vi "Main.vi"(8 "error in":errorcluster, 9 "Error Queue":refnum<queue>, 10 "Controller Queue":refnum<queue>, 11 "Application Events":refnum<user-event>) -> (0 "error out":errorcluster)   [LabVIEW 2020, in "Display Console.lvlib"]
uses:
  Display Console.lvlib
  Controller/Controls/Module Message.ctl
  Controller/Controls/Application Modules.ctl
  Controller/Controls/Application Event Message.ctl
  Controller/Controls/Application Events.ctl
  Controls/Module Loop Data.ctl
  Controller/Controller.lvlib
panel:
  out "Emergency":bool
  out "Door Open":bool
  out "Elevator Direction":cluster{"Up":bool, "Down":bool}
  out "Elevator Location":string
  out "Timing":string
  # "[Covers: UI3] \n[Covers: UI3A] \n[Covers: UI3A1] \n[Covers: UI3A2] \n[Covers: UI3B] \n[Covers: UI3C] \n[Covers: UI3D] \n[Covers: UI3D1] \n[Covers: UI3D2] \n[Covers: UI3E]"
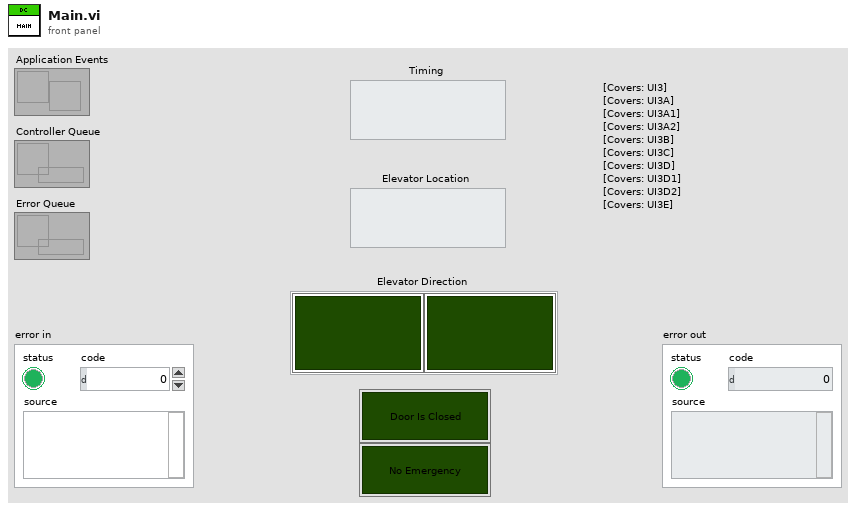
[diagram p1: front panel]
types:
  T1 = typedef "Controller.lvlib/Application Events.ctl" = enum16{"Controller: Initialize", "Controller: Initialize Start And Move State", "Controller: Initialize Analysis State", "Controller: Initialize Continue Travel State", "Controller: Initialize Stop At Floor", "Controller: Initialize Open And Close Door Sequence", "Controller: Initialize No Request Remaining", "Controller: Initialize Emergency Call", "Controller: Initialize Terminate Process", "Controller: Publish State", "UI: Elevator Call", "UI: Broadcast State", "UI: Next Destination Reached", "UI: Timeout Reached", "UI: Emergency Call", "UI: Terminate State", "UI: Door Opened", "UI: Door Closed", "UI: Floor Reached", "UI: Door About To Close"}
  T2 = typedef "Display Console.lvlib/Module Loop Data.ctl" = cluster{"Timing":cluster{"IsTiming?":bool, "Time Target Sec":dbl, "Time Ticks Ms":i32, "Time Ticks Counter":i32, "Timeout Event":T3}, "Is Elevator Travelling?":bool, "Is Elevator opening Door?":bool}
  T3 = typedef "Controller.lvlib/Application Event Message.ctl" = cluster{"Source":T4, "Event":T1, "Data":variant}
  T4 = typedef "Controller.lvlib/Application Modules.ctl" = enum16{"Controller", "User Console", "Display Console", "Sensor Interface", "Configuration Database", "Error Module"}
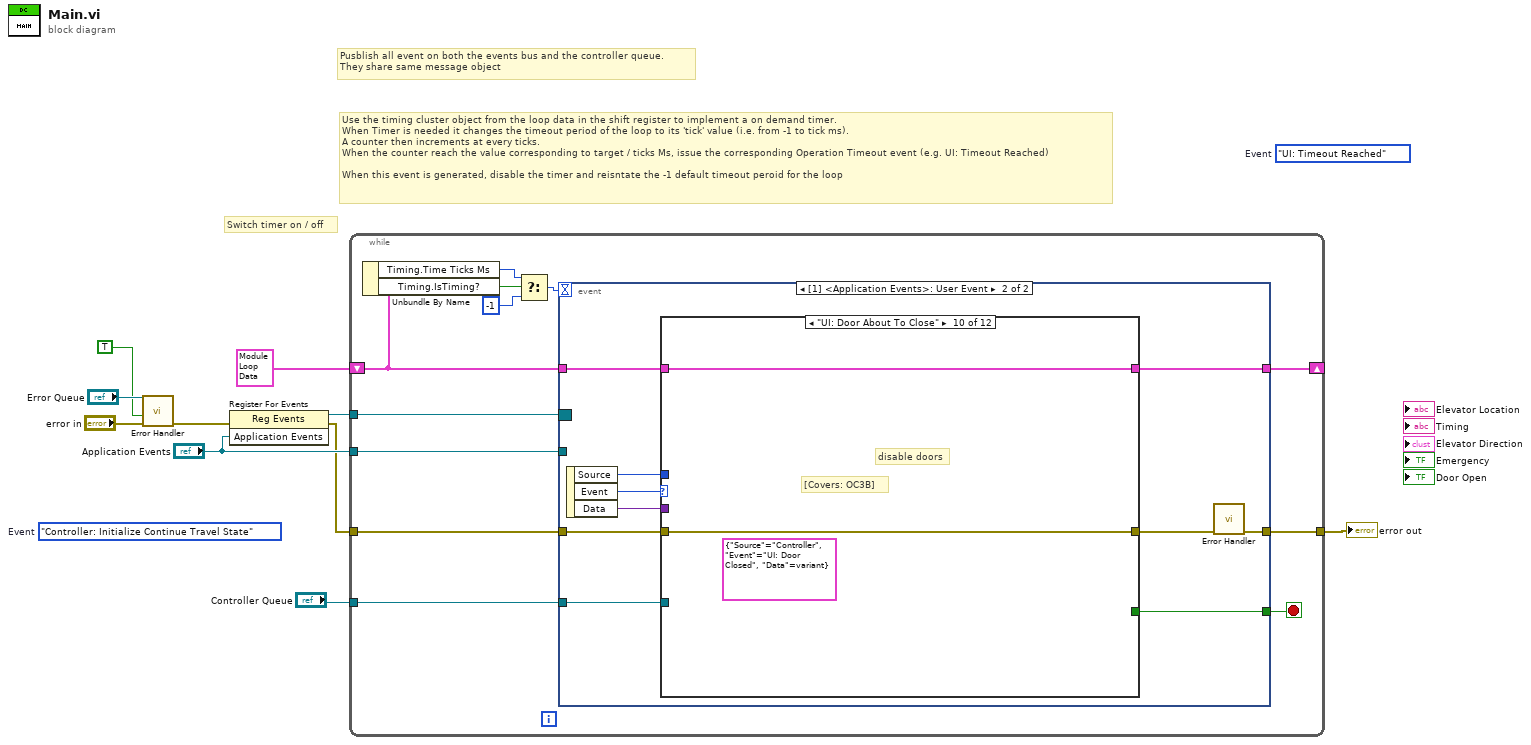
[diagram p0: block diagram]
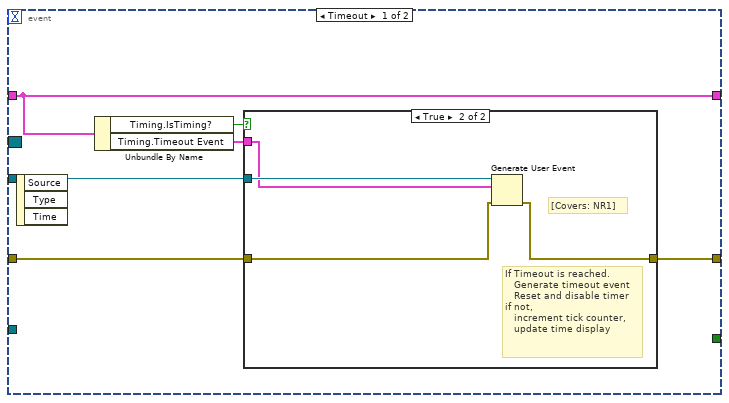
[diagram p2: hidden frame]
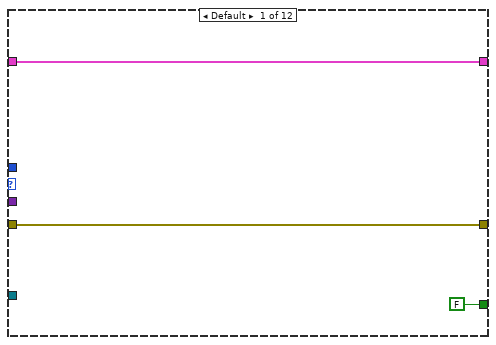
[diagram p4: hidden frame]
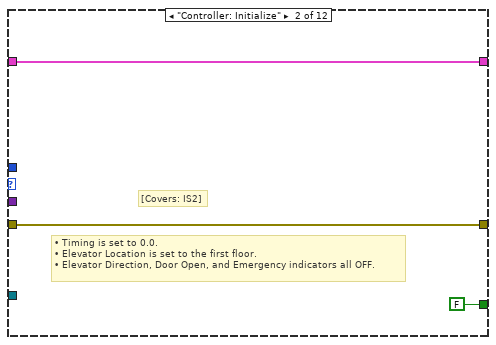
[diagram p5: hidden frame]
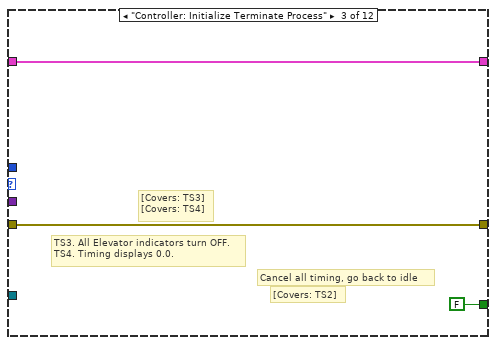
[diagram p6: hidden frame]
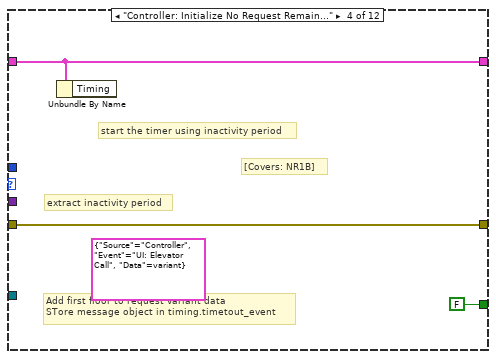
[diagram p7: hidden frame]
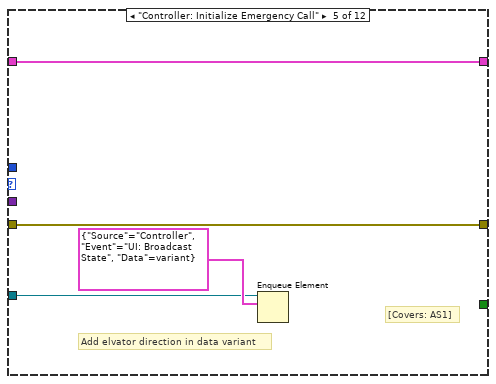
[diagram p8: hidden frame]
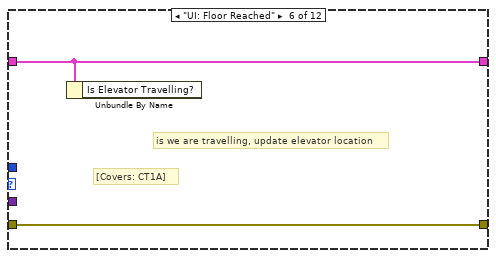
[diagram p9: hidden frame]
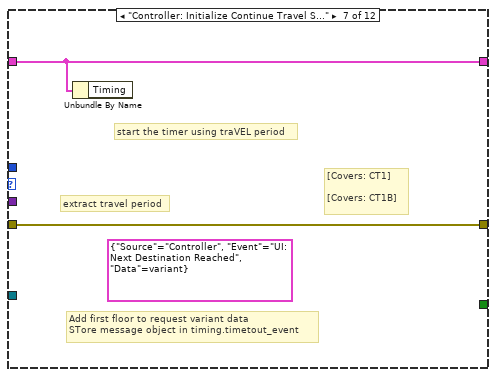
[diagram p10: hidden frame]
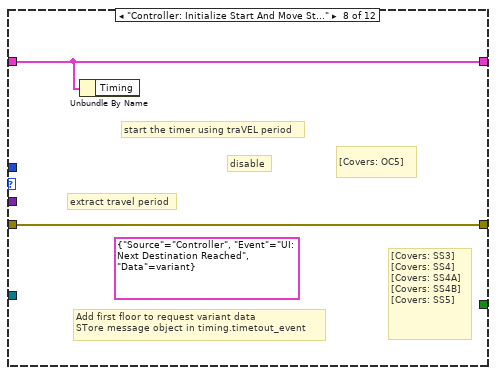
[diagram p11: hidden frame]
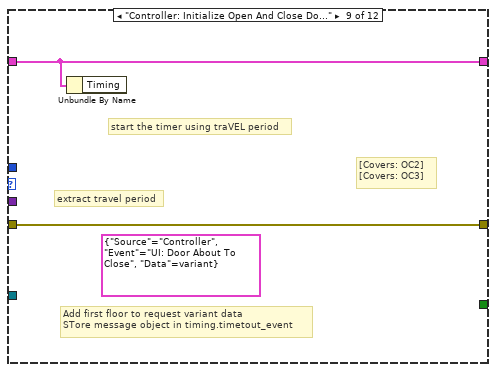
[diagram p12: hidden frame]
diagram:
  (unwired) Application_Events."UI: Timeout Reached"  # Event
  (unwired) Application_Events."Controller: Initialize Continue Travel State"  # Event
  # "Pusblish all event on both the events bus and the controller queue. \nThey share same message object"
  # "Switch timer on / off"
  # "Use the timing cluster object from the loop data in the shift register to implement a on demand timer.\nWhen Timer is needed it changes the timeout period of the loop to its 'tick' value (i.e. from -1 to tick ms). \nA counter then increments at every ticks. \nWhen the counter reach the value corresponding to target / ticks Ms, issue the corresponding Operation Timeout event (e.g. UI: Timeout Reached)\n\nWhen this event is generated, disable the timer and reisntate the -1 default timeout peroid for the loop"
  n1 = call "Error Handler.vi"("error in"="error in", "Load Reference?"=TRUE, "Error Queue"="Error Queue") -> ("error out"=w4:errorcluster)  [unwired: 8 in]
  n2 = register-events(error in=w4, "Application Events") -> (reference out=w9:refnum<event-registration>, error out=w3:errorcluster)  [unwired: 1 in]
  n3 = while {
    tunnel: "Application Events" -> [w22]
    tunnel: w9 -> [w21]
    tunnel: w3 -> [w20]
    tunnel: "Controller Queue" -> [w19]
    tunnel: [w17] -> w2
    shift-right: [w16] -> _
    shift-left: T2 {"Timing"={"IsTiming?"=FALSE, "Time Target Sec"=0.0, "Time Ticks Ms"=0, "Time Ticks Counter"=0, "Timeout Event"={"Source"=enum."Display Console", "Event"=enum."UI: Timeout Reached", "Data"=variant}}, "Is Elevator Travelling?"=FALSE, "Is Elevator opening Door?"=FALSE} ("Event Loop Data") -> [w15]
    stop <- w18 stop-if-true
    n4 = Unbundle By Name(w15) -> ("Timing.Time Ticks Ms"=w11:i32, "Timing.IsTiming?"=w14:bool)
    n5 = Select(t=w11, s=w14, f=-1) -> (s? t:f=w12:i32)
    n6 = event shown="[1] <Application Events>: User Event" {
      selector: w21 -> [_ _]
      dyn-events: _ -> [_ _]
      timeout: w12 -> [_ _]
      tunnel: w22 -> [w27 _]
      tunnel: w20 -> [w26 w38]
      tunnel: w19 -> [_ w34]
      tunnel: [_ w40] -> w18
      tunnel: [w25 w37] -> w17
      tunnel: [w28 w36] -> w16
      tunnel: w15 -> [w28 w35]
      event Timeout {
        n7 = event-data() -> ()  [unwired: 1 in, 3 out]
        n8 = Unbundle By Name(w28) -> ("Timing.IsTiming?"=w24:bool, "Timing.Timeout Event"=w23:T3)
        n9 = case shown="True" w24 {
          tunnel: w27 -> [_ w33]
          tunnel: w26 -> [w29 w32]
          tunnel: [w29 w31] -> w25
          tunnel: w23 -> [_ w30]
          frame False {
          }
          frame True {
            # "If Timeout is reached.\n   Generate timeout event \n   Reset and disable timer\nif not, \n   increment tick counter, \n   update time display"
            # "[Covers: NR1]"
            n10 = Generate User Event(user event=w33, event data cluster=w30, error in=w32) -> (error out=w31:errorcluster)  [unwired: 1 in, 1 out]
          }
        }
      }
      event User Event {
        n11 = event-data() -> ("Source"=w42:T4, "Event"=w43:T1, "Data"=w41:variant)  [unwired: 1 in]
        n12 = case shown="\"UI: Door About To Close\"" w43 {
          tunnel: w42 -> [_ _ _ _ _ _ _ _ _ _ _ _]
          tunnel: w41 -> [_ _ _ _ _ _ _ _ _ _ _ _]
          tunnel: [FALSE FALSE FALSE FALSE _ _ _ _ _ _ _ _] -> w40
          tunnel: [w45 w48 w51 w54 w59 w61 w63 w65 w67 w69 w71 w73] -> w39
          tunnel: w38 -> [w45 w48 w51 w54 w59 w61 w63 w65 w67 w69 w71 w73]
          tunnel: [w44 w47 w50 w53 w58 w60 w62 w64 w66 w68 w70 w72] -> w36
          tunnel: w35 -> [w44 w47 w50 w53 w58 w60 w62 w64 w66 w68 w70 w72]
          tunnel: w34 -> [_ _ _ _ w56 _ _ _ _ _ _ _]
          frame Default {
          }
          frame "Controller: Initialize" {
            # "[Covers: IS2]"
            # "• Timing is set to 0.0.\n• Elevator Location is set to the first floor.\n• Elevator Direction, Door Open, and Emergency indicators all OFF."
          }
          frame "Controller: Initialize Terminate Process" {
            # "Cancel all timing, go back to idle"
            # "[Covers: TS2]"
            # "[Covers: TS3] \n[Covers: TS4]"
            # "TS3. All Elevator indicators turn OFF.\nTS4. Timing displays 0.0."
          }
          frame "Controller: Initialize No Request Remaining" {
            (unwired) T3 {"Source"=enum."Controller", "Event"=enum."UI: Elevator Call", "Data"=variant} ("Timeout Event")
            # "[Covers: NR1B]"
            # "Add first floor to request variant data\nSTore message object in timing.timetout_event"
            # "extract inactivity period"
            # "start the timer using inactivity period"
            n13 = Unbundle By Name(w53) -> ()  [unwired: 1 out]
          }
          frame "Controller: Initialize Emergency Call" {
            # "[Covers: AS1]"
            # "Add elvator direction in data variant"
            n14 = Enqueue Element(queue=w56, element=T3 {"Source"=enum."Controller", "Event"=enum."UI: Broadcast State", "Data"=variant}) -> ()  [unwired: 2 in, 3 out]
          }
          frame "UI: Floor Reached" {
            # "[Covers: CT1A]"
            # "is we are travelling, update elevator location"
            n15 = Unbundle By Name(w60) -> ()  [unwired: 1 out]
          }
          frame "Controller: Initialize Continue Travel State" {
            (unwired) T3 {"Source"=enum."Controller", "Event"=enum."UI: Next Destination Reached", "Data"=variant} ("Timeout Event")
            # "[Covers: CT1] \n\n[Covers: CT1B]"
            # "Add first floor to request variant data\nSTore message object in timing.timetout_event"
            # "extract travel period"
            # "start the timer using traVEL period"
            n16 = Unbundle By Name(w62) -> ()  [unwired: 1 out]
          }
          frame "Controller: Initialize Start And Move State" {
            (unwired) T3 {"Source"=enum."Controller", "Event"=enum."UI: Next Destination Reached", "Data"=variant} ("Timeout Event")
            # "[Covers: OC5]"
            # "disable"
            # "Add first floor to request variant data\nSTore message object in timing.timetout_event"
            # "extract travel period"
            # "start the timer using traVEL period"
            # "[Covers: SS3] \n[Covers: SS4] \n[Covers: SS4A] \n[Covers: SS4B] \n[Covers: SS5]"
            n17 = Unbundle By Name(w64) -> ()  [unwired: 1 out]
          }
          frame "Controller: Initialize Open And Close Door Sequence" {
            (unwired) T3 {"Source"=enum."Controller", "Event"=enum."UI: Door About To Close", "Data"=variant} ("Timeout Event")
            # "[Covers: OC2] \n[Covers: OC3]"
            # "Add first floor to request variant data\nSTore message object in timing.timetout_event"
            # "extract travel period"
            # "start the timer using traVEL period"
            n18 = Unbundle By Name(w66) -> ()  [unwired: 1 out]
          }
          frame "UI: Door About To Close" {
            (unwired) T3 {"Source"=enum."Controller", "Event"=enum."UI: Door Closed", "Data"=variant} ("Timeout Event")
            # "[Covers: OC3B]"
            # "disable doors"
          }
          frame "UI: Door Opened" {
            # "[Covers: OC3A]"
            # "restart timer if doors are opening"
          }
          frame "UI: Door Closed" {
            # "[Covers: OC4]"
          }
        }
        n19 = call "Error Handler.vi"("error in"=w39) -> ("error out"=w37:errorcluster)  [unwired: 10 in]
      }
    }
  }
  "error out" <- w2
